vi "Main.vi"() -> ()   [LabVIEW 2020]
uses:
  User Events/Controls/UEA_Action.ctl
panel:
  out "Error Out":errorcluster
  in  "Error In":errorcluster
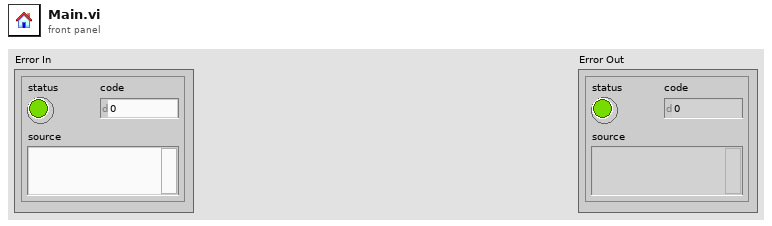
[diagram p1: front panel]
types:
  T1 = typedef "UEA_Action.ctl" = enum16{"Create", "Get", "Destroy"}
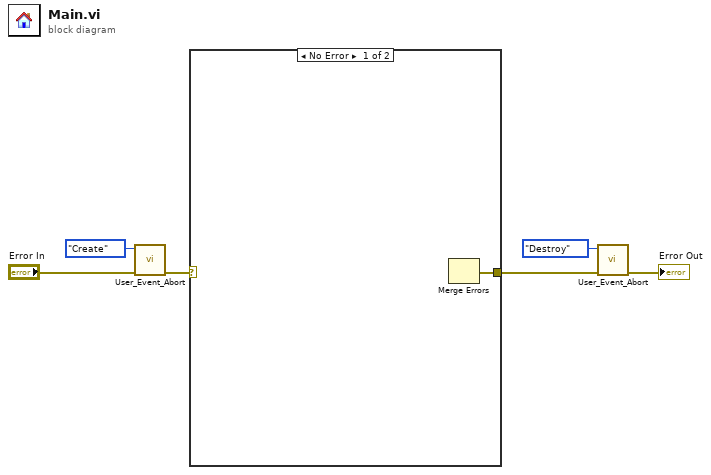
[diagram p0: block diagram]
diagram:
  n1 = call "User_Event_Abort.vi"("Error In"="Error In", "Action"=UEA_Action."Create") -> ("Error Out"=w2:errorcluster)  [unwired: 8 in, 1 out]
  n2 = case shown="No Error" w2 {
    selector: w2 -> [_ w8]
    tunnel: [w7 w8] -> w1
    frame No Error {
      n3 = Merge Errors() -> (w7:errorcluster)  [unwired: 3 in]
    }
    frame Error {
    }
  }
  n4 = call "User_Event_Abort.vi"("Error In"=w1, "Action"=UEA_Action."Destroy") -> ("Error Out"=→"Error Out":errorcluster)  [unwired: 8 in, 1 out]
